vi "Get Temperature WarningLevels.vi"(4 "error in (no error)":errorcluster, 7 "VISA resource name":refnum<visa-resource-name>) -> (0 "error out":errorcluster, 1 "Subtemp (out)":dbl, 2 "Overtemp (out)":dbl, 3 "VISA resource name out":refnum<visa-resource-name>)   [LabVIEW 2018, in "JULABO DeviceDriver.lvlib"]
doc: "This VI returns the warning/alarm levels for Overtemp and Subtemp.\n\nIf for a sensitive temperature application task adherence to a working temperature value <B>Setpoint</B> is to be supervised, then set high and low temperature warning values. In case the internal bath temperature exceeds the specified limits, the instrument will show a warning message or will switch to alarm state depending on the settings in the according menu."
uses:
  JULABO DeviceDriver.lvlib
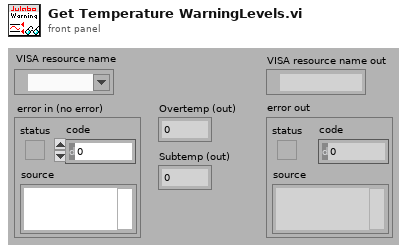
[diagram p1: front panel]
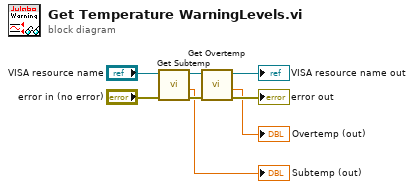
[diagram p0: block diagram]
diagram:
  n1 = call "Get Subtemp.vi"("error in (no error)"="error in (no error)", "VISA resource name"="VISA resource name") -> ("error out"=w3:errorcluster, "Subtemp (out)"=→"Subtemp (out)":dbl, "VISA resource name out"=w4:refnum<visa-resource-name>)  [unwired: 7 in]
  n2 = call "Get Overtemp.vi"("error in (no error)"=w3, "VISA resource name"=w4) -> ("error out"=→"error out":errorcluster, "Overtemp (out)"=→"Overtemp (out)":dbl, "VISA resource name out"=→"VISA resource name out":refnum<visa-resource-name>)  [unwired: 7 in]
